vi "OffsetRect by Point Array and Rect Array.vi"(8 "错误输入":errorcluster, 10 "Points Array":cluster{"x":i16, "y":i16}[](array[cluster])) -> (0 "错误输出":errorcluster, 3 "OffsetRect Array":T1(array[cluster]))   [LabVIEW 2012, in "Picture Box Tools.lvlib" / "Rect Tools.lvlib"]
uses:
  Rect Tools.lvlib
  OffsetRect by Point and Rect.vi
panel:
  in  "Rect Array":T1(array[cluster])
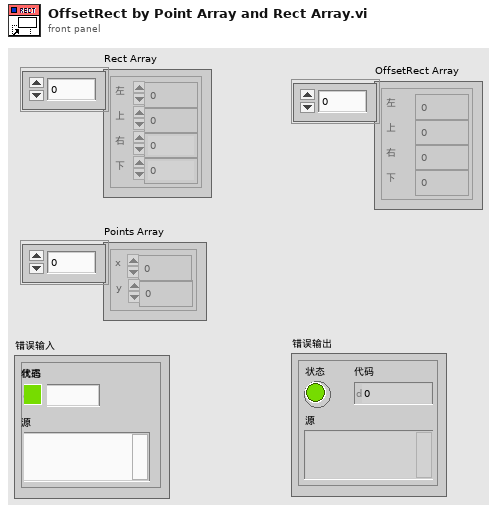
[diagram p1: front panel]
types:
  T1 = cluster{"left":i16, "top":i16, "right":i16, "bottom":i16}[]
  T2 = cluster{"left":i16, "top":i16, "right":i16, "bottom":i16}
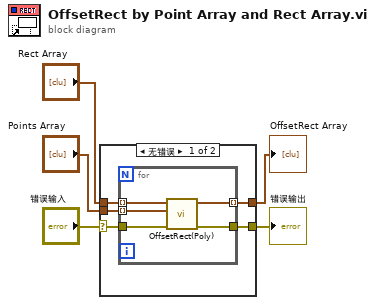
[diagram p0: block diagram]
diagram:
  n1 = case shown="无错误" "错误输入" {
    selector: "错误输入" -> [w8 w16]
    tunnel: [w7 w16] -> w4
    tunnel: [w9 _] -> w2
    tunnel: "Points Array" -> [w10 _]
    tunnel: "Rect Array" -> [w6 _]
    frame No Error {
      n2 = for {
        tunnel: w10 -> [w11] mode=indexing
        tunnel: w6 -> [w15] mode=indexing
        tunnel: [w14] -> w9 mode=indexing
        tunnel: w8 -> [w13]
        tunnel: [w12] -> w7
        n3 = call-poly "OffsetRect(Poly).vi"("错误输入"=w13, "point"=w11, "rect"=w15) -> ("错误输出"=w12:errorcluster, "offset rect"=w14:T2)  [unwired: 7 in]
      }
    }
    frame Error {
    }
  }
  "错误输出" <- w4
  "OffsetRect Array" <- w2
